vi "Main.vi"(8 "Error In":errorcluster) -> (0 "Error Out":errorcluster)   [LabVIEW 2018, in "Controller.lvlib"]
uses:
  Controller.lvlib
  InternalData.ctl
  OracleRequestParameters.ctl
  <vilib>/Utility/file.llb/Read Delimited Spreadsheet (string).vi
  UserEvents/StopUE.lvlib
  ErrorHandler/ErrorHandler.lvlib
panel:
  out "all rows":string[][](array[string])
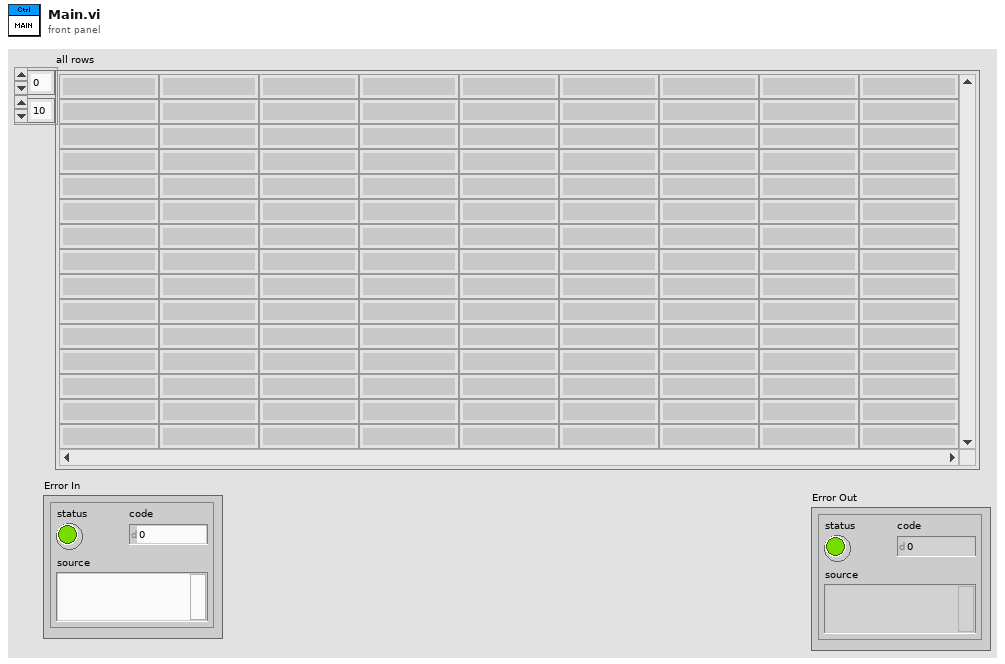
[diagram p1: front panel]
types:
  T1 = typedef "Controller.lvlib/InternalData.ctl" = cluster{"Status":string}
  T2 = cluster{"SRNumber":dbl, "Owner":string, "SRStatus":string, "ProblemDescription":string, "Neglected":bool, "LastUpdate":timestamp}
  T3 = typedef "Controller.lvlib/OracleRequestParameters.ctl" = cluster{"OracleStartDate":timestamp, "OracleEndDate":timestamp, "EmailAddress:":string}
  T4 = typedef "Controller.lvlib/States_Module.ctl" = enum16{"Array2Cluster", "ProcessXLS", "DoSomething", "Shutdown", "Initialize", "RequestOracleReport"}
  T5 = typedef "Controller.lvlib/MessageData.ctl" = cluster{"State":T4, "Payload":variant, "WaitOnReply":bool, "ReplyNotif":refnum<notifier>}
  T6 = cluster{"SRNumber":dbl, "Owner":string, "SRStatus":string, "ProblemDescription":string, "Neglected":bool, "LastUpdate":timestamp}[]
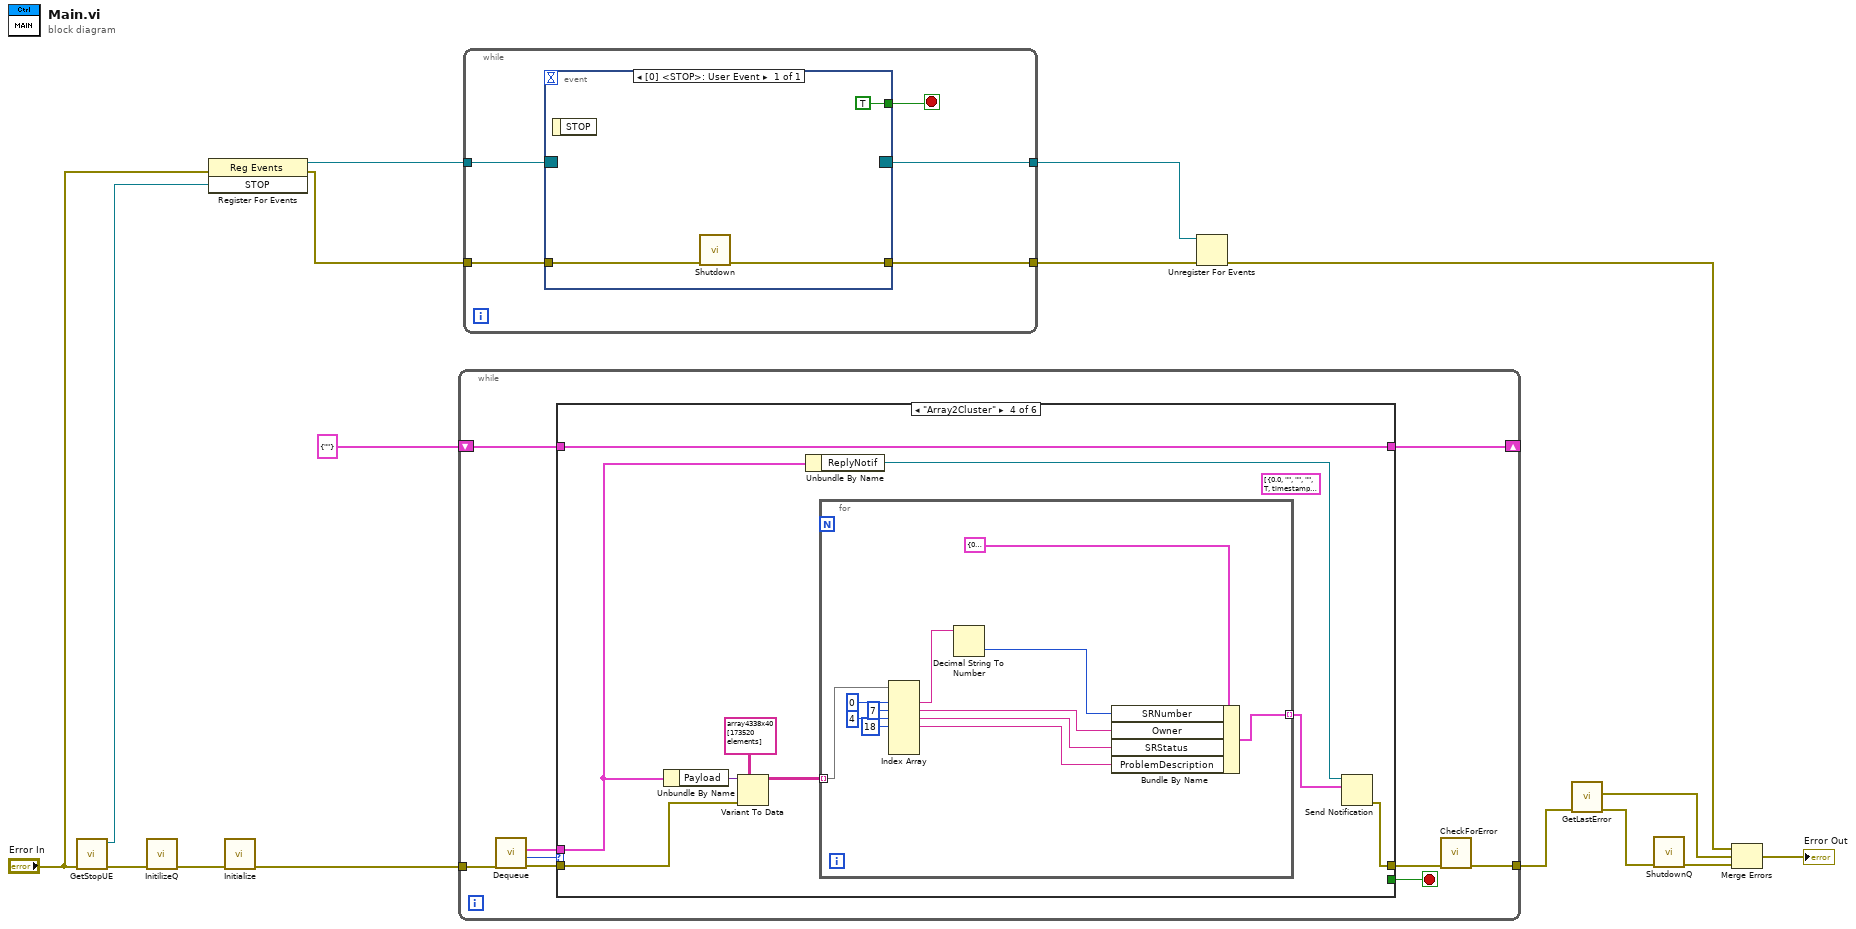
[diagram p0: block diagram]
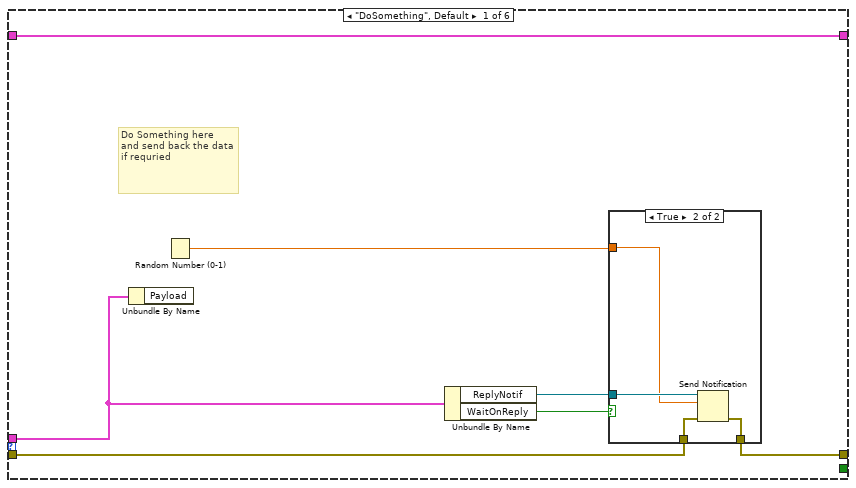
[diagram p2: hidden frame]
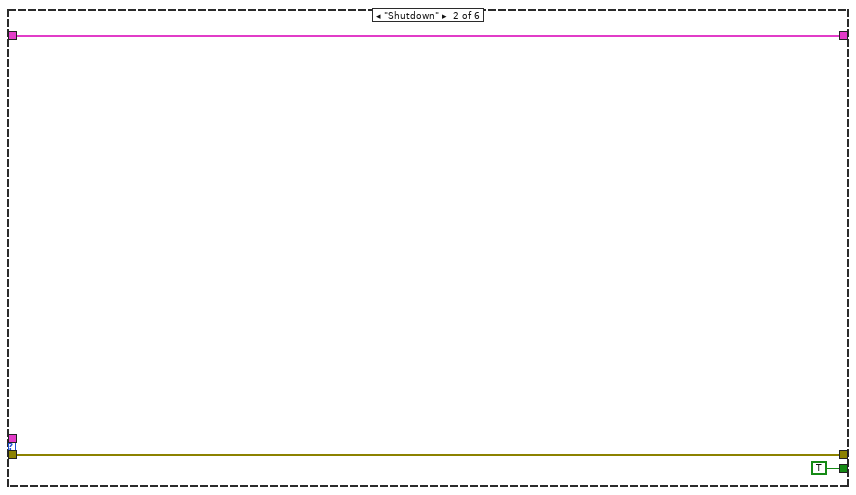
[diagram p4: hidden frame]
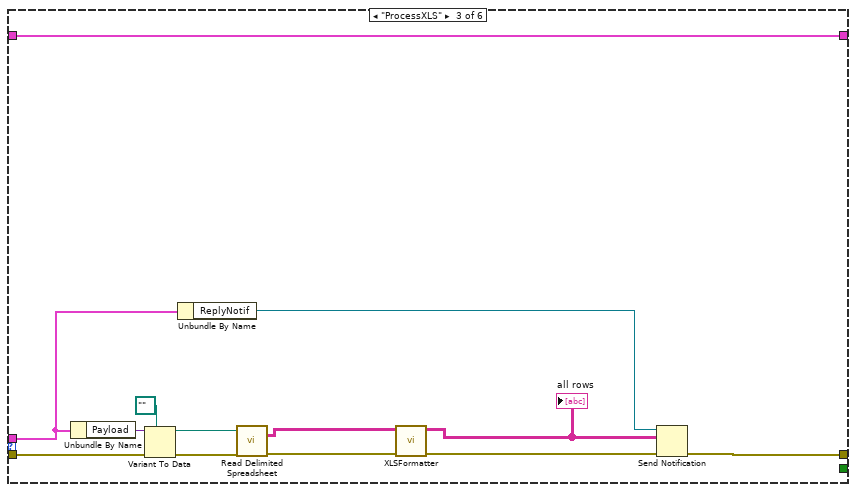
[diagram p5: hidden frame]
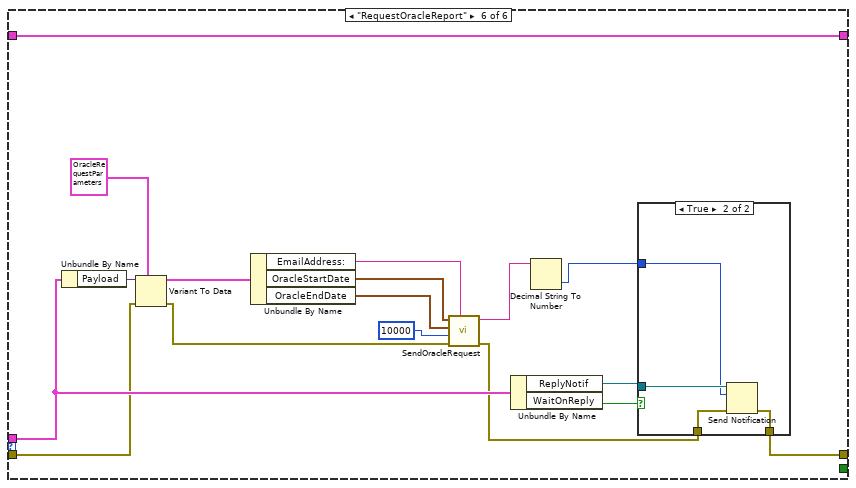
[diagram p7: hidden frame]
diagram:
  n1 = call "GetStopUE.vi"("Error In"="Error In") -> ("Error Out"=w13:errorcluster, "STOP"=w16:refnum<user-event>)  [unwired: 9 in]
  n2 = call "InitilizeQ.vi"("Error In"=w13) -> ("Error Out"=w11:errorcluster)  [unwired: 10 in]
  n3 = register-events(error in="Error In", w16) -> (reference out=w15:refnum<event-registration>, error out=w14:errorcluster)  [unwired: 1 in]
  n4 = call "Initialize.vi"("Error In"=w11) -> ("error out"=w10:errorcluster)  [unwired: 9 in, 1 out]
  n5 = while {
    tunnel: w10 -> [w25]
    tunnel: [w18] -> w7
    shift-right: [w20] -> _
    shift-left: T1 {"Status"=""} ("InternalData") -> [w21]
    stop <- w22 stop-if-true
    n6 = call "Dequeue.vi"("Error In"=w25) -> ("error out"=w24:errorcluster, "State"=w23:T4, "Data out"=w17:T5)  [unwired: 8 in]
    n7 = case shown="\"Array2Cluster\"" w23 {
      tunnel: w24 -> [w31 w39 w51 w59 w76 w86]
      tunnel: [_ TRUE _ _ _ _] -> w22
      tunnel: [w30 w39 w45 w56 w76 w89] -> w19
      tunnel: w21 -> [w32 w38 w53 w62 w75 w93]
      tunnel: [w32 w38 w53 w62 w75 w93] -> w20
      tunnel: w17 -> [w28 _ w48 w58 _ w92]
      frame "DoSomething", Default {
        # "Do Something here\nand send back the data if requried"
        n8 = Unbundle By Name(w28) -> ()  [unwired: 1 out]
        n9 = Random Number (0-1)() -> (number: 0 to 1=w29:dbl)
        n10 = Unbundle By Name(w28) -> ("ReplyNotif"=w26:refnum<notifier>, "WaitOnReply"=w27:bool)
        n11 = case shown="True" w27 {
          tunnel: w31 -> [w33 w37]
          tunnel: [w33 w36] -> w30
          tunnel: w26 -> [_ w35]
          tunnel: w29 -> [_ w34]
          frame False {
          }
          frame True {
            n12 = Send Notification(notification=w34, notifier=w35, error in (no error)=w37) -> (error out=w36:errorcluster)  [unwired: 1 out]
          }
        }
      }
      frame "Shutdown" {
      }
      frame "ProcessXLS" {
        n13 = Unbundle By Name(w48) -> ("Payload"=w52:variant)
        n14 = Variant To Data(error in=w51, type=path "", Variant=w52) -> (data=w49:path, error out=w46:errorcluster)
        n15 = Unbundle By Name(w48) -> ("ReplyNotif"=w47:refnum<notifier>)
        n16 = call-poly <vilib>:"Read Delimited Spreadsheet.vi"("file path (dialog if empty)"=w49, "error in (no error)"=w46) -> ("all rows"=w44:string[][], "error out"=w43:errorcluster)  [unwired: 8 in, 4 out]
        n17 = call "XLSFormatter.vi"("error in (no error)"=w43, "Array"=w44) -> ("error out"=w42:errorcluster, "Array 2"=w41:string[][])  [unwired: 8 in]
        "all rows" <- w41
        n18 = Send Notification(notification=w41, notifier=w47, error in (no error)=w42) -> (error out=w45:errorcluster)  [unwired: 1 out]
      }
      frame "Array2Cluster" {
        (unwired) T6 [{"SRNumber"=0.0, "Owner"="", "SRStatus"="", "ProblemDescription"="", "Neglected"=TRUE, "LastUpdate"=timestamp(0 s since 1904-01-01)}, {"SRNumber"=0.0, "Owner"="", "SRStatus"="", "ProblemDescription"="", "Neglected"=TRUE, "LastUpdate"=timestamp(0 s since 1904-01-01)}, {"SRNumber"=0.0, "Owner"="", "SRStatus"="", "ProblemDescription"="", "Neglected"=TRUE, "LastUpdate"=timestamp(0 s since 1904-01-01)}, {"SRNumber"=0.0, "Owner"="", "SRStatus"="", "ProblemDescription"="", "Neglected"=TRUE, "LastUpdate"=timestamp(0 s since 1904-01-01)}, {"SRNumber"=0.0, "Owner"="", "SRStatus"="", "ProblemDescription"="", "Neglected"=TRUE, "LastUpdate"=timestamp(0 s since 1904-01-01)}, {"SRNumber"=0.0, "Owner"="", "SRStatus"="", "ProblemDescription"="", "Neglected"=TRUE, "LastUpdate"=timestamp(0 s since 1904-01-01)}, {"SRNumber"=0.0, "Owner"="", "SRStatus"="", "ProblemDescription"="", "Neglected"=FALSE, "LastUpdate"=timestamp(0 s since 1904-01-01)}] ("SR_Cluster")
        n19 = Unbundle By Name(w58) -> ("Payload"=w61:variant)
        n20 = Variant To Data(error in=w59, type=string[][] array4338x40[173520 elements] ("all rows"), Variant=w61) -> (data=w55:string[][])  [unwired: 1 out]
        n21 = Unbundle By Name(w58) -> ("ReplyNotif"=w60:refnum<notifier>)
        n22 = for {
          tunnel: w55 -> [w74] mode=indexing
          tunnel: [w72] -> w54 mode=indexing
          n23 = Index Array(array=w74, index #1=0, index #2=7 ("index"), index #3=4 ("index"), index #4=18 ("index")) -> (element #1=w69:string, element #2=w67:string, element #3=w65:string, element #4=w64:string)  [unwired: 3 in, 3 out]
          n24 = Decimal String To Number(string=w69) -> (number=w70:i32)  [unwired: 2 in, 1 out]
          n25 = Bundle By Name(cluster=T2 {"SRNumber"=0.0, "Owner"="", "SRStatus"="", "ProblemDescription"="", "Neglected"=FALSE, "LastUpdate"=timestamp(0 s since 1904-01-01)} ("Cluster"), "SRNumber"=w70, "Owner"=w67, "SRStatus"=w65, "ProblemDescription"=w64) -> (w72:T2)
        }
        n26 = Send Notification(notification=w54, notifier=w60) -> (error out=w56:errorcluster)  [unwired: 1 in, 1 out]
      }
      frame "Initialize" {
      }
      frame "RequestOracleReport" {
        n27 = Unbundle By Name(w92) -> ("Payload"=w88:variant)
        n28 = Variant To Data(error in=w86, type=T3 {"OracleStartDate"=timestamp(0 s since 1904-01-01), "OracleEndDate"=timestamp(0 s since 1904-01-01), "EmailAddress:"=""} ("cluster"), Variant=w88) -> (data=w87:T3, error out=w84:errorcluster)
        n29 = Unbundle By Name(w87) -> ("EmailAddress:"=w77:string, "OracleStartDate"=w80:timestamp, "OracleEndDate"=w79:timestamp)
        n30 = call "SendOracleRequest.vi"("Email"=w77, "error in (no error)"=w84, "Timeout"=10000, "Report End Date"=w79, "Report Start Date"=w80) -> ("error out"=w83:errorcluster, "String"=w81:string)  [unwired: 5 in]
        n31 = Unbundle By Name(w92) -> ("ReplyNotif"=w91:refnum<notifier>, "WaitOnReply"=w90:bool)
        n32 = Decimal String To Number(string=w81) -> (number=w78:i32)  [unwired: 2 in, 1 out]
        n33 = case shown="True" w90 {
          tunnel: [w94 w98] -> w89
          tunnel: w91 -> [_ w97]
          tunnel: w78 -> [_ w96]
          tunnel: w83 -> [w94 w95]
          frame False {
          }
          frame True {
            n34 = Send Notification(notification=w96, notifier=w97, error in (no error)=w95) -> (error out=w98:errorcluster)  [unwired: 1 out]
          }
        }
      }
    }
    n35 = call "CheckForError.vi"("Error In"=w19) -> ("error out"=w18:errorcluster)  [unwired: 10 in]
  }
  n36 = while {
    tunnel: w15 -> [w103]
    tunnel: w14 -> [w101]
    tunnel: [w100] -> w9
    tunnel: [w99] -> w8
    stop <- w102 stop-if-true
    n37 = event shown="[0] <STOP>: User Event" {
      selector: w103 -> [_]
      dyn-events: [_] -> w99
      timeout: _ -> [_]
      tunnel: [TRUE] -> w102
      tunnel: w101 -> [w105]
      tunnel: [w104] -> w100
      event User Event {
        n38 = event-data() -> ()  [unwired: 1 in, 1 out]
        n39 = call "Shutdown.vi"("Error In"=w105) -> ("error out"=w104:errorcluster)  [unwired: 9 in, 1 out]
      }
    }
  }
  n40 = Unregister For Events(event registration refnum=w8, error in=w9) -> (error out=w3:errorcluster)
  n41 = call "GetLastError.vi"("Error In"=w7) -> ("error IO"=w6:errorcluster, "Last Error"=w4:errorcluster)  [unwired: 9 in]
  n42 = call "ShutdownQ.vi"("Error In"=w6) -> ("Error Out"=w5:errorcluster)  [unwired: 10 in]
  n43 = Merge Errors(w3, w4, w5) -> (→"Error Out":errorcluster)
